vi "Stop All Displays dialog.vi"(11 "Displays":refnum<class "Message Enqueuer.lvclass">[](array[class])) -> ()   [LabVIEW 2016, in "Assert API Components.lvlib" / "Assert Startup UI.lvlib" / "Assert Startup UI.lvclass"]
uses:
  Assert Startup UI.lvclass
  <vilib>/ActorFramework/Message Enqueuer/Message Enqueuer.lvclass
  <vilib>/ActorFramework/Message Enqueuer/Message Enqueuer.lvclass/Message Enqueuer.ctl
  <vilib>/ActorFramework/Message Enqueuer/Enqueue.vi
  <vilib>/ActorFramework/Stop Msg/Stop Msg.lvclass
  C:/Program Files (x86)/National Instruments/LabVIEW 2016/vi.lib/ActorFramework/Message/Message.lvclass
  <vilib>/ActorFramework/Message Priority Queue/Priority Enqueue.vi
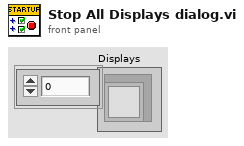
[diagram p1: front panel]
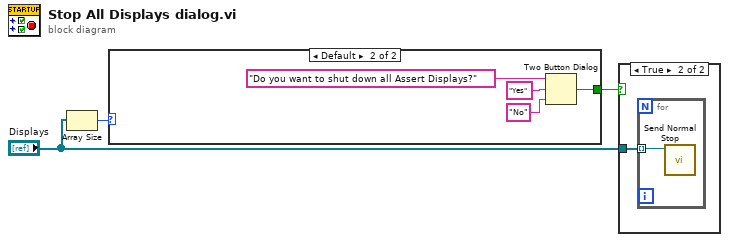
[diagram p0: block diagram]
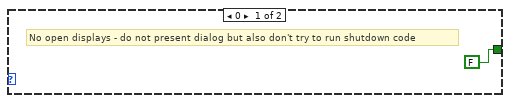
[diagram p3: hidden frame]
diagram:
  n1 = Array Size(array="Displays") -> (size(s)=w3:i32)
  n2 = case shown="Default" w3 {
    tunnel: [FALSE ("T button?") w8] -> w2
    frame 0 {
      # "No open displays - do not present dialog but also don't try to run shutdown code"
    }
    frame Default {
      n3 = Two Button Dialog(message="Do you want to shut down all Assert Displays?", 1:"No" ("F button name (\"Cancel\")"), 2:"Yes" ("T button name (\"OK\")")) -> (T button?=w8:bool)
    }
  }
  n4 = case shown="True" w2 {
    tunnel: "Displays" -> [_ w9]
    frame False {
    }
    frame True {
      n5 = for {
        tunnel: w9 -> [w10] mode=indexing
        n6 = call <vilib>:"Send Normal Stop.vi"("Message Enqueuer"=w10) -> ()  [unwired: 10 in, 1 out]
      }
    }
  }
